vi "Create Server Message Queues.vi"(8 "error in (no error)":errorcluster) -> (0 "error out":errorcluster, 3 "Message Queues Out":T1)   [LabVIEW 2024, in "Message Queue.lvlib"]
doc: "Creates and initializes the client message queues for your application. If your application requires more message queues, right-click the \"Message Queues\" constant above and select Open Type Def. Add the new message queues to the type definition, then initialize them in this VI."
uses:
  Message Queue.lvlib
  Server Message Queues.ctl
  Message Cluster.ctl
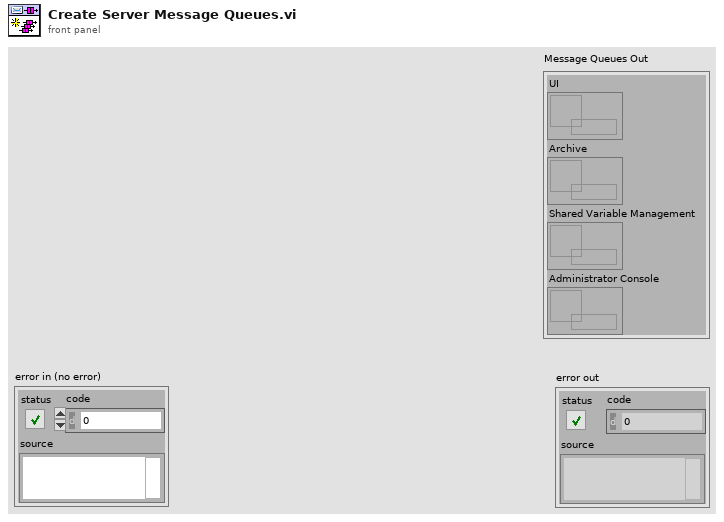
[diagram p1: front panel]
types:
  T1 = typedef "Message Queue.lvlib/Server Message Queues.ctl" = cluster{"UI":refnum<queue>, "Archive":refnum<queue>, "Shared Variable Management":refnum<queue>, "Administrator Console":refnum<queue>}
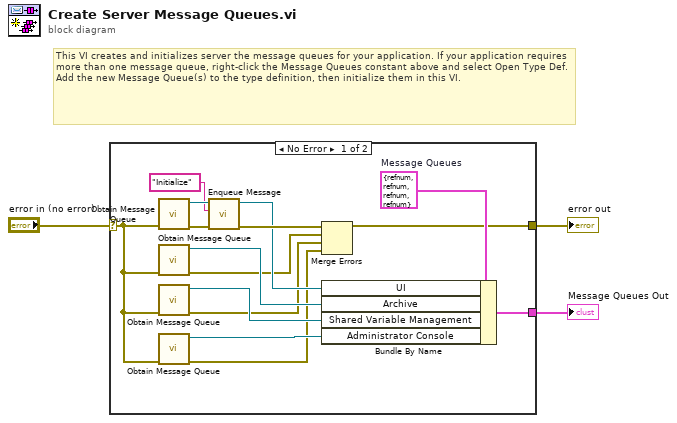
[diagram p0: block diagram]
diagram:
  # "This VI creates and initializes server the message queues for your application. If your application requires more than one message queue, right-click the Message Queues constant above and select Open Type Def.  Add the new Message Queue(s) to the type definition, then initialize them in this VI."
  n1 = case shown="No Error" "error in (no error)" {
    selector: "error in (no error)" -> [w4 w19]
    tunnel: [w13 w19] -> w3
    tunnel: [w16 _] -> w1
    frame No Error {
      w17 = T1 {"UI"=refnum, "Archive"=refnum, "Shared Variable Management"=refnum, "Administrator Console"=refnum}  # Message Queues
      n2 = call "Obtain Message Queue.vi"("error in (no error)"=w4) -> ("error out"=w15:errorcluster, "Message Queue"=w14:refnum<queue>)  [unwired: 9 in]
      n3 = call "Obtain Message Queue.vi"("error in (no error)"=w4) -> ("error out"=w9:errorcluster, "Message Queue"=w11:refnum<queue>)  [unwired: 9 in]
      n4 = call "Obtain Message Queue.vi"("error in (no error)"=w4) -> ("error out"=w8:errorcluster, "Message Queue"=w10:refnum<queue>)  [unwired: 9 in]
      n5 = call "Obtain Message Queue.vi"("error in (no error)"=w4) -> ("error out"=w5:errorcluster, "Message Queue"=w6:refnum<queue>)  [unwired: 9 in]
      n6 = call "Enqueue Message.vi"("error in (no error)"=w15, "Message"="Initialize", "Message Queue"=w14) -> ("error out"=w18:errorcluster, "dup Message Queue"=w12:refnum<queue>)  [unwired: 7 in]
      n7 = Merge Errors(w18, w9, w8, w5) -> (w13:errorcluster)
      n8 = Bundle By Name(cluster=w17, "UI"=w12, "Archive"=w11, "Shared Variable Management"=w10, "Administrator Console"=w6) -> (w16:T1)
    }
    frame Error {
    }
  }
  "Message Queues Out" <- w1
  "error out" <- w3
